vi "CopyCrossCorrelationResult.vi"(2 "tracker":u64) -> (3 "x prof":sgl[](array[numeric]), 4 "y prof":sgl[](array[numeric]), 5 "tracker":u64, 7 "x result":sgl[](array[numeric]), 8 "y_result":sgl[](array[numeric]))   [LabVIEW 2011]
uses:
  TrackerDLL.vi
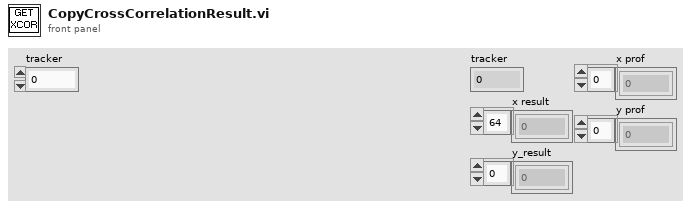
[diagram p1: front panel]
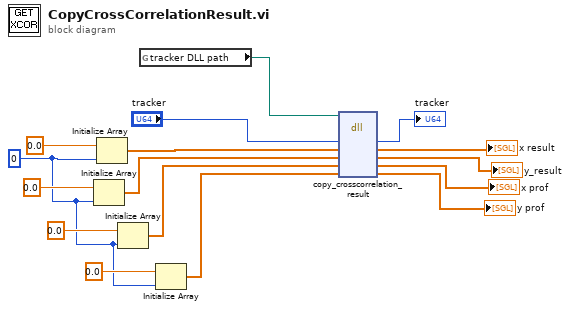
[diagram p0: block diagram]
diagram:
  w1 = 0 ("dimension size")
  n1 = Initialize Array(sgl 0.0 ("element"), w1) -> (w9:sgl[])
  n2 = Initialize Array(sgl 0.0 ("element"), w1) -> (w11:sgl[])
  n3 = Initialize Array(sgl 0.0 ("element"), w1) -> (w6:sgl[])
  n4 = global read "TrackerDLL.vi" "tracker DLL path"() -> (w16:path)
  n5 = Initialize Array(sgl 0.0 ("element"), w1) -> (w5:sgl[])
  n6 = dll-call lib="?" fn="copy_crosscorrelation_result"(path in=w16, "tracker"="tracker", "x_result"=w11, "y_result"=w9, "x_xc"=w6, "y_xc"=w5) -> ("tracker"=→"tracker":u64, "x_result"=→"x result":sgl[], "y_result"=→"y_result":sgl[], "x_xc"=→"x prof":sgl[], "y_xc"=→"y prof":sgl[])  [unwired: 3 in, 2 out]
